vi "AOI to optional rectangle.vi"(4 "x1, y1, x2, y2 with origin (0, 0)":u16[](array[numeric]) caption="Aoi in") -> (1 "x1, y1, x2+1, y2+1 with origin (0, 0)":u16[](array[numeric]) caption="Optional rectangle out", 2 "Rectangle Out":T1)   [LabVIEW 2011]
doc: "This conversion is required by the semi-insane way that NI defines the \"optional rectangle\" input of IMAQ ImageToArray. If the input parameter is empty, the output will be empty."
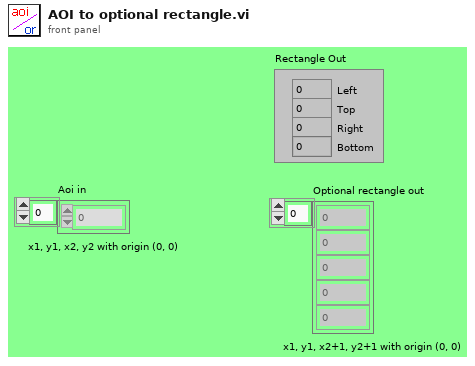
[diagram p1: front panel]
types:
  T1 = cluster{"Left":i32, "Top":i32, "Right":i32, "Bottom":i32}
  T2 = cluster{"x1, y1, x2, y2 with origin (0, 0)[0]":u16, "x1, y1, x2, y2 with origin (0, 0)[1]":u16, "x1, y1, x2, y2 with origin (0, 0)[2]":u16, "x1, y1, x2, y2 with origin (0, 0)[3]":u16, "x1, y1, x2, y2 with origin (0, 0)[4]":u16, "x1, y1, x2, y2 with origin (0, 0)[5]":u16, "x1, y1, x2, y2 with origin (0, 0)[6]":u16, "x1, y1, x2, y2 with origin (0, 0)[7]":u16, "x1, y1, x2, y2 with origin (0, 0)[8]":u16}
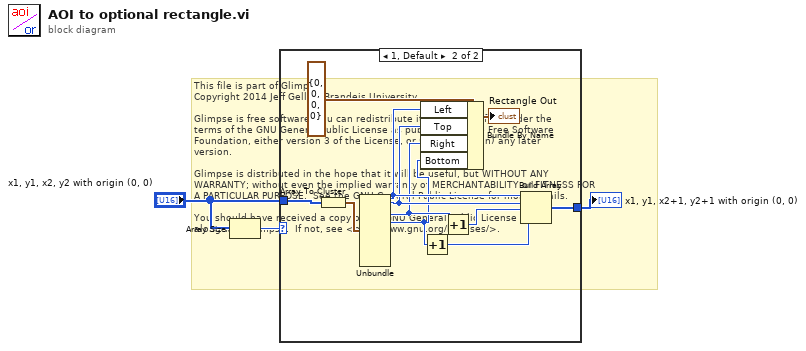
[diagram p0: block diagram]
diagram:
  # "This file is part of Glimpse. \nCopyright 2014 Jeff Gelles, Brandeis University.    \n\nGlimpse is free software: you can redistribute it and/or modify it under the \nterms of the GNU General Public License as published by the Free Software \nFoundation, either version 3 of the License, or (at your option) any later \nversion.\n\nGlimpse is distributed in the hope that it will be useful, but WITHOUT ANY \nWARRANTY; without even the implied warranty of MERCHANTABILITY or FITNESS FOR \nA PARTICULAR PURPOSE.  See the GNU General Public License for more details.\n\nYou should have received a copy of the GNU General Public License\nalong with Glimpse.  If not, see <http://www.gnu.org/licenses/>."
  n1 = Array Size(array="x1, y1, x2, y2 with origin (0, 0)") -> (size(s)=w1:i32)
  n2 = case shown="1, Default" w1 {
    tunnel: "x1, y1, x2, y2 with origin (0, 0)" -> [w4 w15]
    tunnel: [w4 w11] -> w3
    frame 0 {
    }
    frame 1, Default {
      n3 = Array To Cluster(array=w15) -> (cluster=w14:T2)
      n4 = Unbundle(w14) -> ("x1, y1, x2, y2 with origin (0, 0)[0]"=w8:u16, "x1, y1, x2, y2 with origin (0, 0)[1]"=w7:u16, "x1, y1, x2, y2 with origin (0, 0)[2]"=w6:u16, "x1, y1, x2, y2 with origin (0, 0)[3]"=w5:u16)  [unwired: 5 out]
      n5 = Bundle By Name(cluster=T1 {"Left"=0, "Top"=0, "Right"=0, "Bottom"=0} ("Rectangle Out"), "Left"=w8, "Top"=w7, "Right"=w6, "Bottom"=w5) -> (→"Rectangle Out":T1)
      n6 = Increment(x=w5) -> (x+1=w12:u16)
      n7 = Increment(x=w6) -> (x+1=w13:u16)
      n8 = Build Array(w8, w7, w13, w12) -> (w11:u16[])
    }
  }
  "x1, y1, x2+1, y2+1 with origin (0, 0)" <- w3
